vi "Get Output.vi"(8 "error in (no error)":errorcluster, 11 "Rover in":refnum<class "Rover.lvclass">) -> (0 "error out":errorcluster, 2 "Outputs":T1, 3 "Rover out":refnum<class "Rover.lvclass">)   [LabVIEW 2020, in "Rover.lvlib" / "Rover.lvclass"]
uses:
  Rover.lvclass
  Outputs.ctl
  I2C Register.ctl
  Rover.lvclass/Rover.ctl
  <vilib>/MakerHub/LINX/Private/Local IO/LinxI2cWrite.vi
  <vilib>/MakerHub/LINX/Public/Utilities/Check Channel.vi
  <vilib>/MakerHub/LINX/Private/Local IO/Handle Errors.vi
  <vilib>/MakerHub/LINX/Private/Utilties/Generate Error.vi
  <vilib>/MakerHub/LINX/LMH-LINX.lvlib
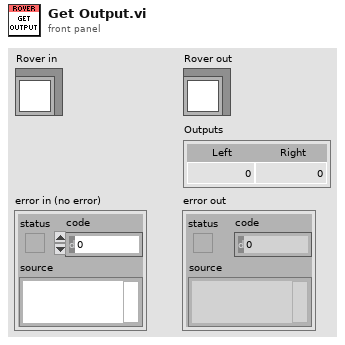
[diagram p1: front panel]
types:
  T1 = typedef "Rover.lvlib/Rover.lvclass/Outputs.ctl" = cluster{"Left":i16, "Right":i16}
  T2 = typedef "Rover.lvlib/Rover.lvclass/I2C Register.ctl" = enum8{"encA", "encB", "ticksPerUnit", "width", "flags", "velP", "velI", "velD", "velMin", "velMax", "poseX", "poseY", "poseA", "cmdDrive", "cmdTurn", "velocity", "turn", "velL", "velR", "run", "outL", "outR", "outDeadband"}
  T3 = typedef "LMH-LINX.lvlib/LINX Ref.ctl" = cluster{"IO":T4, "Interface":T5, "LINX Device Config":T6}
  T4 = typedef "LMH-LINX.lvlib/Platform.ctl" = enum16{"Remote", "Local"}
  T5 = typedef "LMH-LINX.lvlib/Interface.ctl" = enum16{"Serial", "TCP"}
  T6 = typedef "LMH-LINX.lvlib/Device.lvlib/LINX Device Config.ctl" = cluster{"Interface":T5, "COM Port":refnum<visa-resource-name>, "TCP Configuration":T7, "Device Family":u8, "Device ID":u8, "Device Name":string, "TCP Ref":refnum<k5>, "Channels":T8}
  T7 = typedef "LMH-LINX.lvlib/Device.lvlib/TCP Config.ctl" = cluster{"IP Address":string, "Port":u16}
  T8 = typedef "LMH-LINX.lvlib/Channels.ctl" = cluster{"DI":u8[], "DO":u8[], "AI":u8[], "AO":u8[], "PWM":u8[], "QE":u8[], "UART":u8[], "I2C 2":u8[], "SPI":u8[], "CAN":u8[], "Servo":u8[], "AI Ref (V)":dbl, "AI Resolution (Bits)":u8, "AO Ref (V)":dbl, "AO Resolution (Bits)":u8}
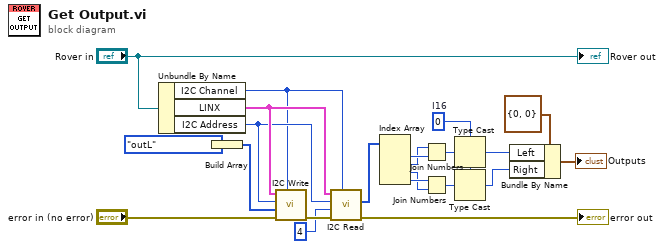
[diagram p0: block diagram]
diagram:
  w2 = i16 0  # I16
  n1 = Unbundle By Name("Rover in") -> ("I2C Channel"=w18:u8, "LINX"=w20:T3, "I2C Address"=w19:u8)
  n2 = Build Array(I2C_Register."outL" ("I2C Register")) -> (w22:T2[])
  n3 = call <vilib>:"I2C Write.vi"("I2C Channel"=w18, "Error In"="error in (no error)", "Data"=w22, "I2C Slave Address (0)"=w19, "LINX Resource"=w20) -> ("Error Out"=w21:errorcluster)  [unwired: 5 in, 1 out]
  n4 = call <vilib>:"I2C Read.vi"("I2C Channel"=w18, "Error In"=w21, "Bytes To Read"=u8 4, "I2C Slave Address (0)"=w19, "LINX Resource"=w20) -> ("Error Out"=→"error out":errorcluster, "Data"=w10:u8[])  [unwired: 4 in, 1 out]
  n5 = Index Array(array=w10) -> (element #1=w9:u8, element #2=w8:u8, element #3=w3:u8, element #4=w4:u8)  [unwired: 4 in]
  n6 = Join Numbers(hi=w8, lo=w9) -> ((hi.lo)=w7:u16)
  n7 = Join Numbers(hi=w4, lo=w3) -> ((hi.lo)=w5:u16)
  n8 = Type Cast(type=w2, x=w7) -> (*(type *) &x=w6:i16)
  n9 = Type Cast(type=w2, x=w5) -> (*(type *) &x=w1:i16)
  n10 = Bundle By Name(cluster=T1 {"Left"=0, "Right"=0} ("Outputs"), "Left"=w6, "Right"=w1) -> (→"Outputs":T1)
  "Rover out" <- "Rover in"
